vi "Interpolate Complex.vi"(0 "Z":cdb[](array[numeric]), 2 "n":dbl[](array[numeric]), 3 "interpolation_degree":i32=1, 4 "method":i32(ring)=2 items=["nearest", "linear", "spline", "cubic Hermite", "Lagrange"]) -> (7 "Z_interpolated":cdb[](array[numeric]), 9 "n_interpolated":dbl[](array[numeric]), 10 "N_interpolated":i32)   [LabVIEW 2014]
uses:
  <vilib>/gmath/NI_Gmath.lvlib
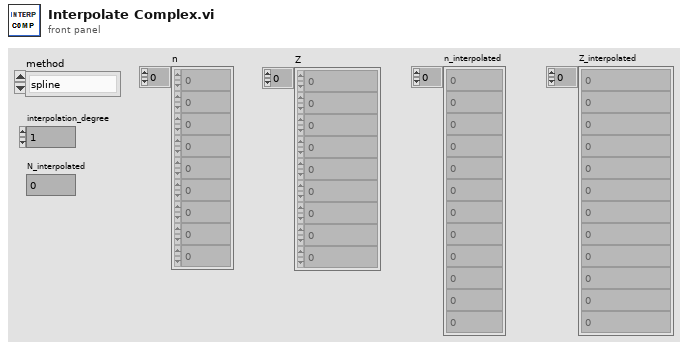
[diagram p1: front panel]
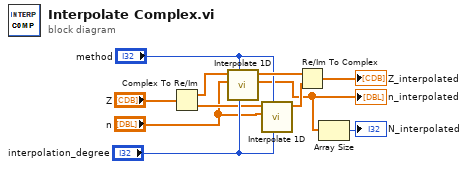
[diagram p0: block diagram]
diagram:
  n1 = Complex To Re/Im(x + iy="Z") -> (x=w11:dbl[], y=w2:dbl[])
  n2 = call <vilib>:"Interpolate 1D.vi"("ntimes"="interpolation_degree", "method"="method", "X"="n", "Y"=w11) -> ("xi used"=w4:dbl[], "yi"=w7:dbl[])  [unwired: 5 in, 1 out]
  "n_interpolated" <- w4
  n3 = call <vilib>:"Interpolate 1D.vi"("ntimes"="interpolation_degree", "method"="method", "X"="n", "Y"=w2) -> ("yi"=w8:dbl[])  [unwired: 5 in, 2 out]
  n4 = Re/Im To Complex(1:w8, 2:w7) -> (0:→"Z_interpolated":cdb[])
  n5 = Array Size(array=w4) -> (size(s)=→"N_interpolated":i32)
